vi "Write State.vi"(8 "error in (no error)":errorcluster, 10 "State":enum16{"Exit", "Kick", "DefBallPos", "GoToBall"}(ring), 11 "DefendAreaTacticVSS in":refnum<class "DefendAreaTacticVSS.lvclass">) -> (0 "error out":errorcluster, 3 "DefendAreaTacticVSS out":refnum<class "DefendAreaTacticVSS.lvclass">)   [LabVIEW 2020, in "DefendAreaTacticVSS.lvclass"]
uses:
  DefendAreaTacticVSS.lvclass
  DefendAreaTacticVSS.lvclass/DefendAreaTacticVSS.ctl
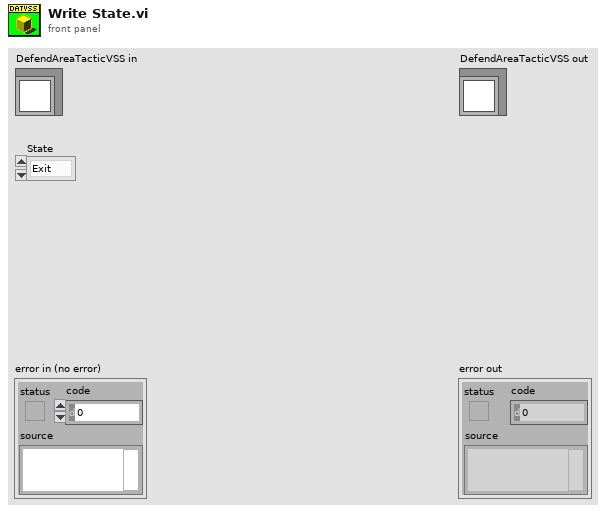
[diagram p1: front panel]
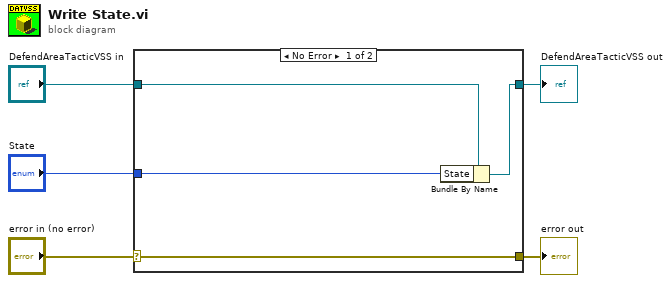
[diagram p0: block diagram]
diagram:
  n1 = case shown="No Error" "error in (no error)" {
    selector: "error in (no error)" -> [w9 w10]
    tunnel: [w9 w10] -> w4
    tunnel: [w7 w11] -> w2
    tunnel: "DefendAreaTacticVSS in" -> [w8 w11]
    tunnel: "State" -> [w6 _]
    frame No Error {
      n2 = Bundle By Name(cluster=w8, "State"=w6) -> (w7:refnum<class "DefendAreaTacticVSS.lvclass">)
    }
    frame Error {
    }
  }
  "error out" <- w4
  "DefendAreaTacticVSS out" <- w2
